vi "Handle Core Error.vi"(8 "error in (no error)":errorcluster, 11 "Interruptible Reply Core in":refnum<class "Interruptible Reply Core.lvclass">) -> (0 "error out":errorcluster, 3 "Interruptible Reply Core out":refnum<class "Interruptible Reply Core.lvclass">)   [LabVIEW 2020, in "Publisher.lvlib" / "Interruptible Reply Core.lvclass"]
doc: "Handle Response Core errors at the end of the Response Msg Send method.\n\nThis implementation removes errors caused by the Drop method."
uses:
  Interruptible Reply Core.lvclass
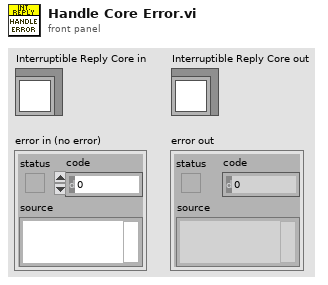
[diagram p1: front panel]
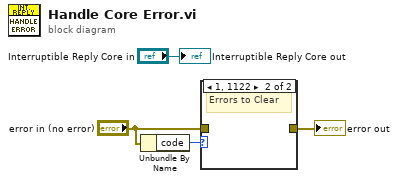
[diagram p0: block diagram]
diagram:
  n1 = Unbundle By Name("error in (no error)") -> ("code"=w3:i32)
  n2 = case shown="1, 1122" w3 {
    tunnel: [w5 _] -> w2
    tunnel: "error in (no error)" -> [w5 _]
    frame Default {
      # "Maintain error"
    }
    frame 1, 1122 {
      # "Errors to Clear"
    }
  }
  "error out" <- w2
  "Interruptible Reply Core out" <- "Interruptible Reply Core in"
